vi "f1.vi"() -> ()   [LabVIEW 2026]
uses:
  <vilib>/Analysis/baseanly.llb/Mean (DBL).vi
  <vilib>/numeric/Random Number (Range) DBL.vi
  <vilib>/Analysis/NI_AALBase.lvlib
panel:
  out "opony":cluster{"laps":i32[], dbl[]}[](graph)
  out "zuzycie":cluster{"laps":i32[], dbl[]}[](graph)
  out "czysty":cluster{"laps":i32[], dbl[]}[](graph)
  out "czas":cluster{"laps":i32[], "times":dbl[]}[](graph)
  in  "Porównanie wybranych kierowców\n 2":bool
  in  "kierowca":i32[](listbox)
  out "Error - graph":string
  out "XY Graph 2":cluster{dbl[], dbl[]}(graph)
  in  "wyświetl mapę":bool
  in  "pobierz_kwalifikacje\n 2":bool
  in  "placement":i32[](listbox)
  in  "gp":i32(listbox)
  in  "sezony":i32(listbox)
  in  "pobierz_sezony":bool
  in  "pobierz_gp":bool
  in  "?":enum32{"Sterowanie"}(tab)
  in  "?":bool
  in  "Module path:":path
  in  "Python path:":path
  # "Zanim włączymy progam należy podać siężkę do pythona (wymagana wersja 3.12.x).\n\n     - dla systemu Windows: <dysk>:\\Users\\<użytkownik>\\AppData\\Local\\Programs\\Python\\Python312\n     - dla systemu Mac: /Library/Frameworks/Python.Frameworks/Versions/3.12\n     - dla systemu Linux: /usr/bin/python3 lub /usr/local/bin/python3\n\nPotrzebne biblioteki Pythona, które należy zainsalować przy pomocy pip (bez tworzenia wirtualnego środowiska):\n\n     - urllib3\n\ngdzie:\n     - <dysk>, oznacza dysk główny, na którym znajduje się system \n     - <użytkownik>, nazwa użytkownika\n\nDodatkowo należy podać ścieżkę do modułu, czyli pliku api_F1.py, który znajduje się w folderze z projektem."
  # "Instrukcja obsługi:\n\n1. Pobieranie sezonów, kliknij przycisk \"Pobierz sezony\" — zostanie załadowana lista dostępnych sezonów F1.\n2. Pobieranie wyścigów GP, wybierz sezon z listy, a następnie kliknij przycisk \"Pobierz GP\" — wyświetli się lista Grand Prix dla danego sezonu. \n3. Pobieranie kwalifikacji, kliknij przycisk \"Pobierz kwalifikacje\" — zostaną wyświetleni kierowcy i ich wyniki z kwalifikacji.\n4. Wyświetlanie mapy toru, kliknij przycisk \"Pokaż mapę wybranego GP\" — na ekranie pojawi się schemat toru.\n\nUwaga: Jeśli mapa dla wybranego wyścigu nie istnieje w bazie danych, wyświetli się komunikat informacyjny pod przyciskiem."
  # "Wyniki wybranej kwalifikacji:"
  # "Skórty w wynikach F1:\nDNF - Did Not Finish: nie ukończył\nDNS - Did Not Stat: nie wystartował\nDSQ - Disqualified: dyskwalifikowany\nNC - Not Classified: nie sklasyfikowany\nDNQ - Did Not Qualify: nie zakwalifikował się\nWD - Withdrawn: wycofał się"
  # "Opis i interpretacja wykresów:\n\nCzas okrążeń ( lewy-górny wykres ): \n        - Co przedstawia: Rzeczywisty czas przejechania każdego okrążenia przez kierowcę (w sekundach)\n        - Jak interpretować:\n                  => Spadki - kierowca przyspiesza (nowe opony, mniej paliwa, czsyte okrążenie)\n                  => Wzrosty - kierowca zwalnia (zużyte opony, ruch na torzem obrona pozycji)\n                  => Nagłe piki w górę - pit stop, Safety Car, Virtual Safety Car lub incydent na torze\n                  => Sawtooth (piła) - typowy wzór przy wieloktrotch pitach\n\nCzas \"czysty\" ( prawy-górny wykres ):\n       - Co przedstawia: czas okrążenia po odjęciu wpływu paliwa i opon - teoretyczny czas kierwocy na \"świeżych oponach i z pustym bakiem\"\n       - Jak interpretować: \n                 => Pozwala ocenić czyste tempo kierowcy bez wpływu strategii\n                 => Spadki - kierowca jedzie coraz szybciej (zyskuje doświadczenie w wyścigu, poprawia linie)\n                 => Wzrosty - kierowca ma problem (ruch na torze, błędy, uszkodzenia)\n                 => Prównanie z rzeczystiwtym czasem - różnica pokazuje, ile stracił przez strategię (paliwo + opony)\n\nZużycie paliwa ( lewy-dolny wykres ):\n       - Co przedstawia: Ilość paliwa pozostałego w baku w każdym momencie wyścigu (w kg)\n       - Jak interpretować: \n                 => Linia malejąca - im mniej paliwa, tym lżejszy bolid\n                 => Małe wahania - różnice w zużyciu wynikające z tempa jazdy (szybciej = więcej paliwa)\n                  \nNotka: Zużycie paliwa jest symulowane na podstawie założonego modelu (start z pełnym bakiem ok. 100L, liniowe lub niemal liniowe zużycie z niewielkimi losowymi wahaniami). Nie są to rzeczywiste dane telemetryczne z bolidu.\n\nZyżycie opon ( prawy-dolny wykres ):\n       - Co przedstawia: skumulowana strata czasowa wynikająca z degreadacji opon (w sekundach)\n       - Jak interpretować: \n                 => Odcinki rosnące - opony się zużywają, bolid traci przyczepność i jest wolniejszy\n                 => Spadki do zera - moment wymiany opon w pit stopie (reset zużycia)\n                 => Nachylenie krzywej - szybkość degradacji (im stromiej, tym szybciej opony tracą przyczepność)\n\nNotka: Zyżycie opon jest symulowane (model liniowy z resetem przy pit stopie). W rzeczywistości degradacja zależy od typu opon, temperatury, stylu jazdy i charakterystyki toru - model upraszcza te zależność do stałej straty na okrążenie"
  # "Jeżeli program przestanie odpowiadać, zatnie się lub nic nie będzie się wyświetlało przez dłuższy czas należy zrestartować projekt."
  # "Uwaga techniczna: W przypadku porównania wielu kierowców każdy kierowca rysowany jest na osobnym plocie. Numer plotu zaczyna się od 0 — plot 0 to pierwszy kierowca, plot 1 to drugi kierowca itd. Property Node Active Plot oraz Plot.Name \nmogą powodować błąd — w około 50% przypadków powodowały błąd Invalid property value (Hex 0x435), niezależnie od ustawienia Plots[].Size. Jeżeli pojawi się błąd z tym związany należy kliknąć \"Continue\" do momentu nieskończenia się powiadomień."
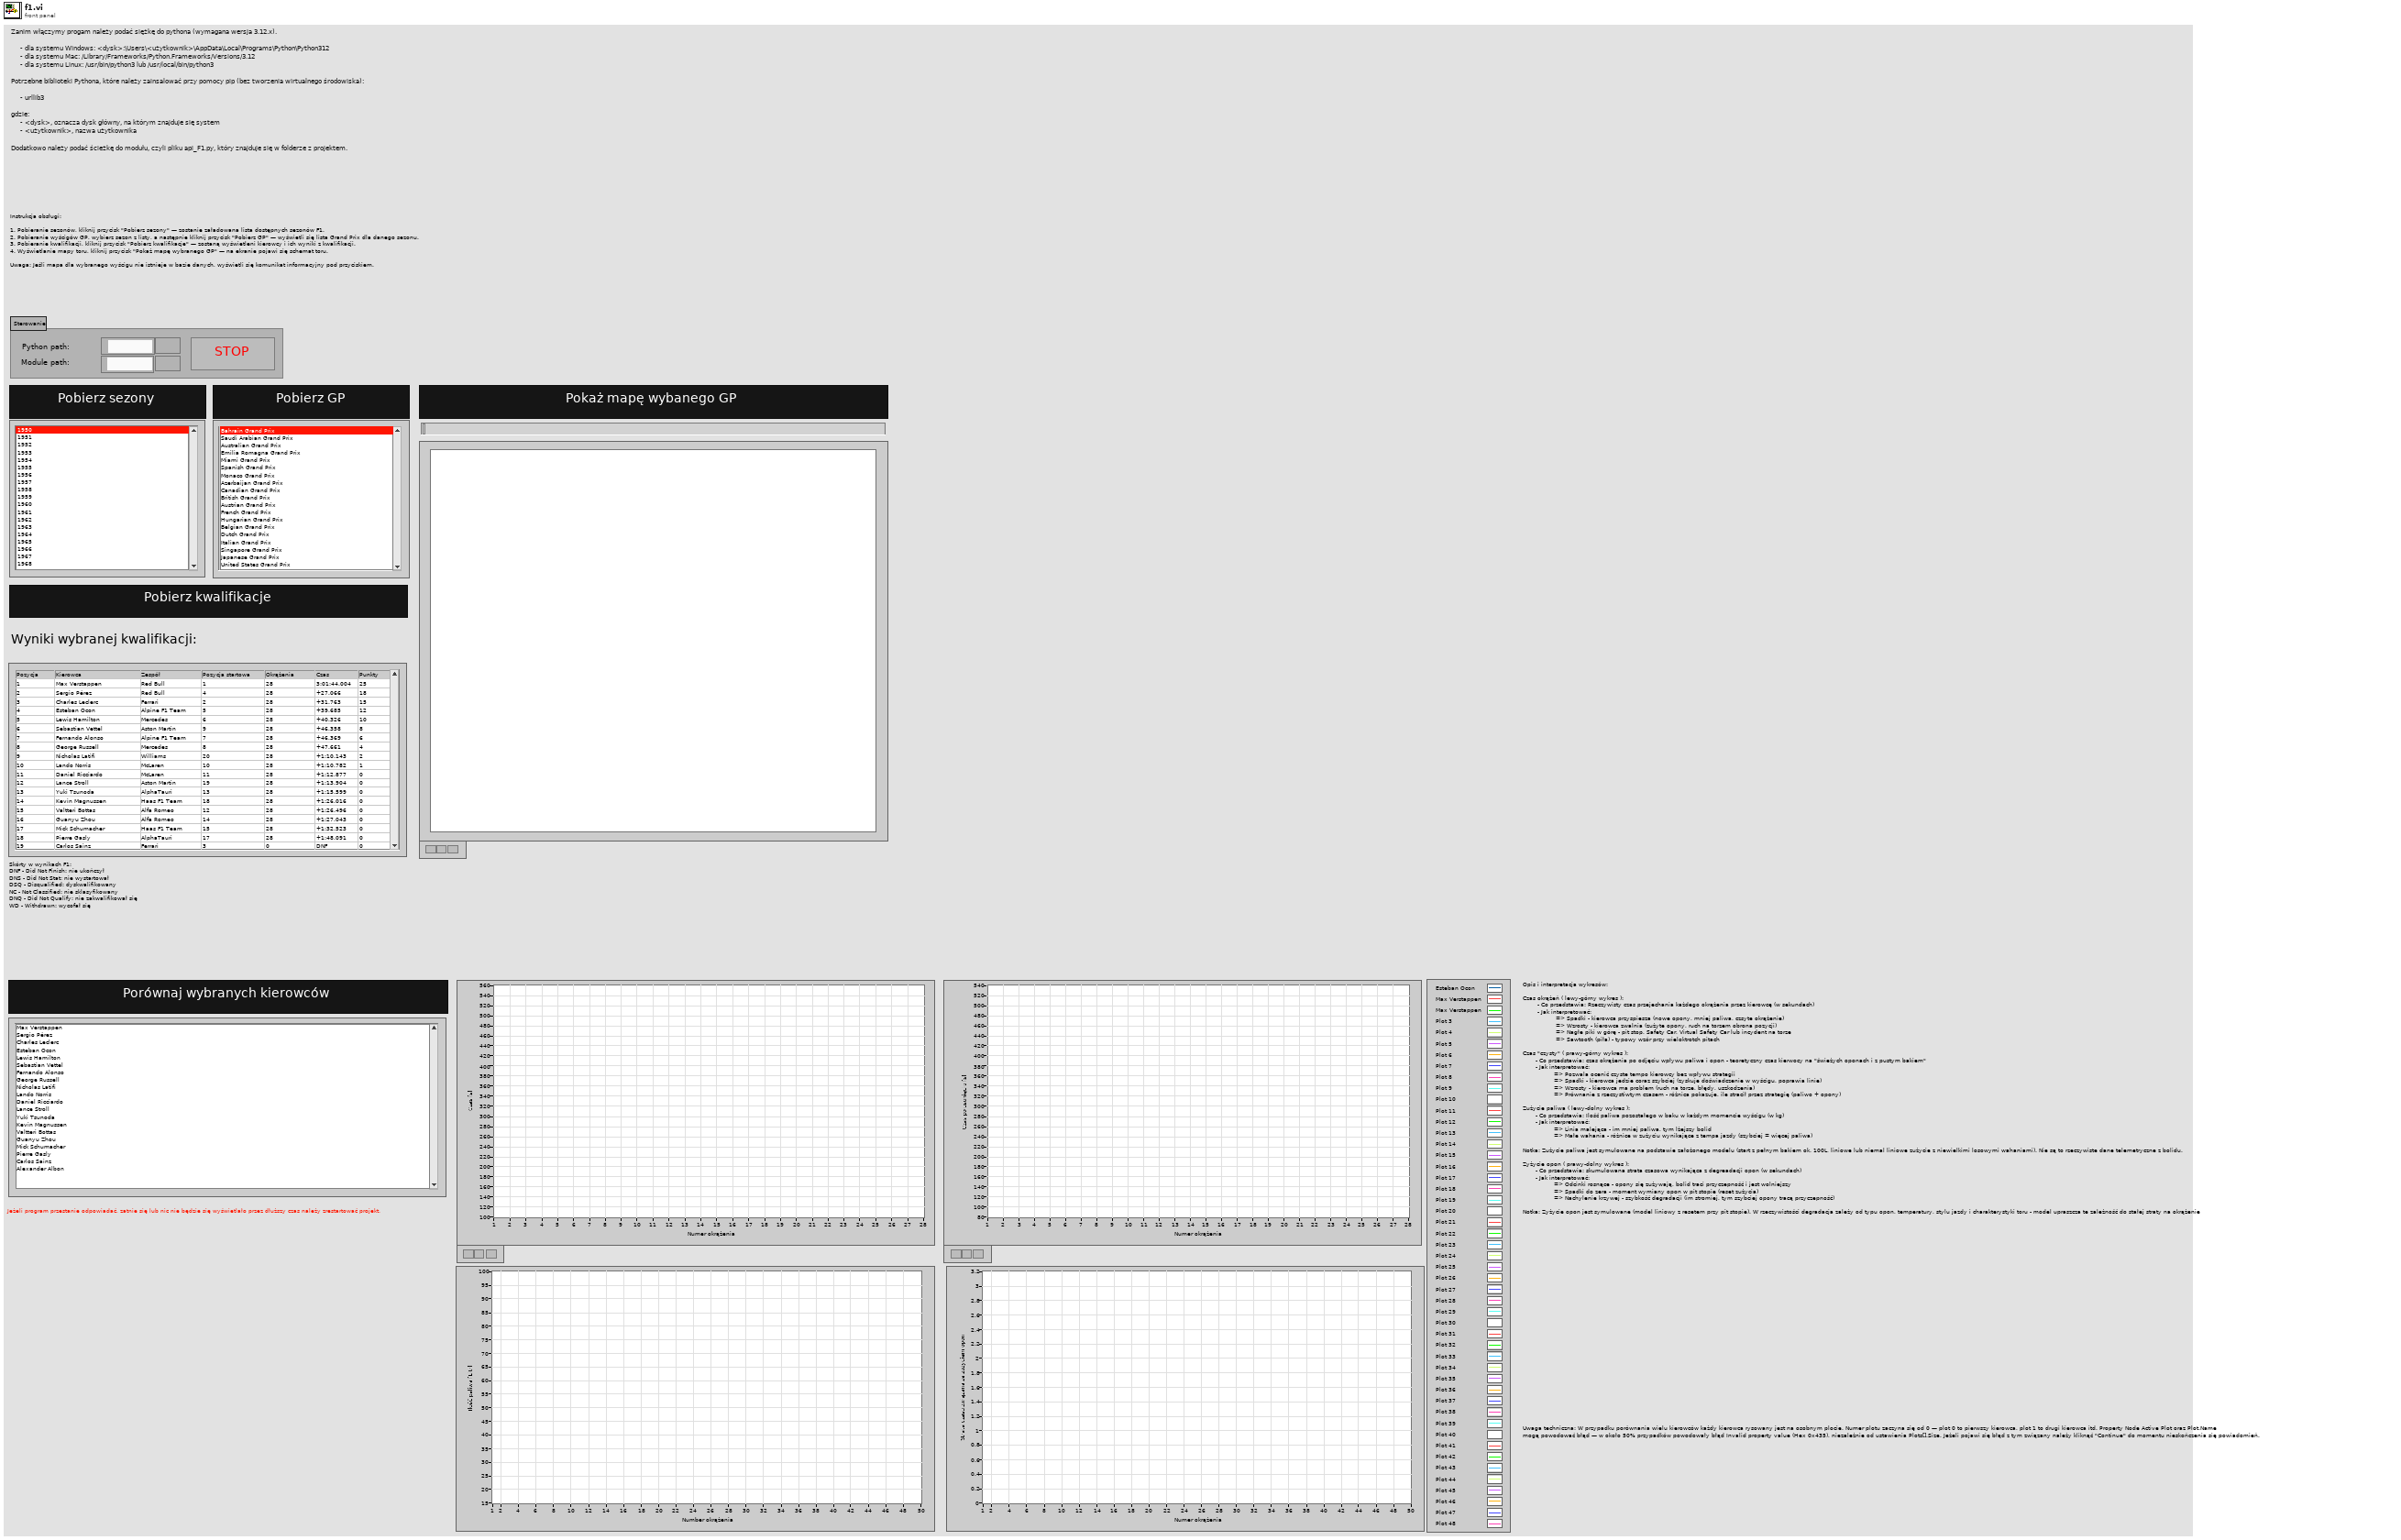
[diagram p1: front panel]
types:
  T1 = cluster{"error":string, "laps":i32[], "times":dbl[], "pits":i32[]}
  T2 = cluster{"position":string, "driver":string, "team":string, "grid":string, "laps":string, "time":string, "points":string}[]
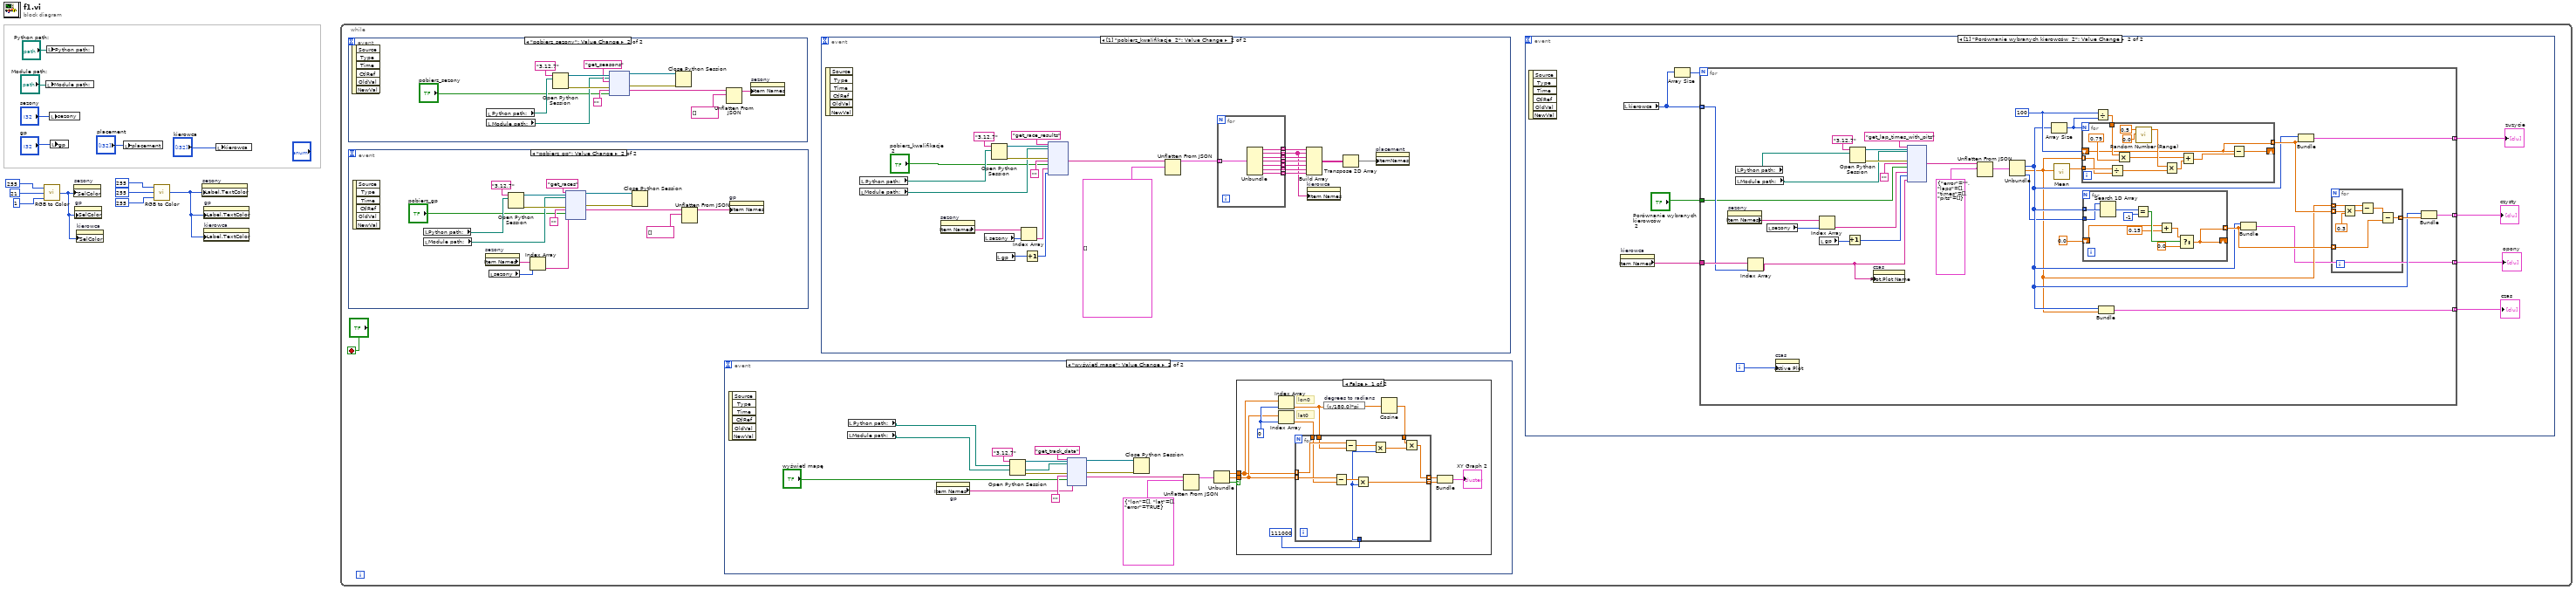
[diagram p0: block diagram]
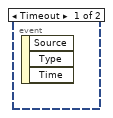
[diagram p2: hidden frame]
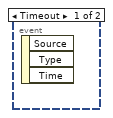
[diagram p3: hidden frame]
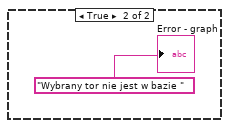
[diagram p4: hidden frame]
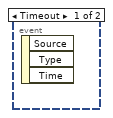
[diagram p5: hidden frame]
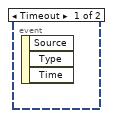
[diagram p6: hidden frame]
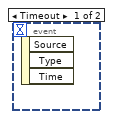
[diagram p7: hidden frame]
diagram:
  n1 = call <vilib>:"RGB to Color.vi"("B"=u8 1, "G"=u8 21, "R"=u8 255) -> ("Color"=w5:u32)
  n2 = local write "Module path:"("Module path:") -> ()
  n3 = local write "Python path:"("Python path:") -> ()
  n4 = local write "sezony"("sezony") -> ()
  n5 = local write "gp"("gp") -> ()
  n6 = property on="sezony" class="LstBox (strict)"("SelColor"=w5) -> ()  [unwired: 2 in, 2 out]
  n7 = property on="gp" class="LstBox (strict)"("SelColor"=w5) -> ()  [unwired: 2 in, 2 out]
  n8 = property on="kierowca" class="LstBox (strict)"("SelColor"=w5) -> ()  [unwired: 2 in, 2 out]
  n9 = local write "placement"("placement") -> ()
  n10 = call <vilib>:"RGB to Color.vi"("B"=u8 255, "G"=u8 255, "R"=u8 255) -> ("Color"=w1:u32)
  n11 = property on="sezony" class="LstBox (strict)"("Label.TextColor"=w1) -> ()  [unwired: 2 in, 2 out]
  n12 = property on="gp" class="LstBox (strict)"("Label.TextColor"=w1) -> ()  [unwired: 2 in, 2 out]
  n13 = property on="kierowca" class="LstBox (strict)"("Label.TextColor"=w1) -> ()  [unwired: 2 in, 2 out]
  n14 = local write "kierowca"("kierowca") -> ()
  n15 = while {
    stop <- "?" stop-if-true
    n16 = event shown="[1] \"pobierz_sezony\": Value Change" {
      selector: _ -> [_ _]
      dyn-events: _ -> [_ _]
      timeout: _ -> [_ _]
      event Timeout {
        n17 = event-data() -> ()  [unwired: 1 in, 3 out]
      }
      event "pobierz_sezony": Value Change {
        n18 = event-data() -> ()  [unwired: 1 in, 6 out]
        n19 = local read "Python path:"() -> (w183:path)
        n20 = local read "Module path:"() -> (w182:path)
        n21 = Open Python Session(python version="3.12.7" ("Python version"), python path=w183) -> (session out=w187:refnum<k35>, error out=w188:errorcluster)  [unwired: 1 in]
        n22 = node ("Python Node")(w187, w182, "get_seasons" ("function name"), w188, "", "pobierz_sezony") -> (w189:refnum<k35>, w190:errorcluster, w178:string)  [unwired: 1 in, 2 out]
        n23 = Close Python Session(session in=w189, error in=w190) -> ()  [unwired: 1 out]
        n24 = Unflatten From JSON(JSON string=w178, type and defaults=string[] []) -> (value=w181:string[])  [unwired: 5 in, 1 out]
        n25 = property on="sezony" class="LstBox (strict)"("Item Names"=w181) -> ()  [unwired: 2 in, 2 out]
      }
    }
    n26 = event shown="[1] \"pobierz_gp\": Value Change" {
      selector: _ -> [_ _]
      dyn-events: _ -> [_ _]
      timeout: _ -> [_ _]
      event Timeout {
        n27 = event-data() -> ()  [unwired: 1 in, 3 out]
      }
      event "pobierz_gp": Value Change {
        n28 = event-data() -> ()  [unwired: 1 in, 6 out]
        n29 = local read "Python path:"() -> (w168:path)
        n30 = local read "Module path:"() -> (w167:path)
        n31 = property on="sezony" class="LstBox (strict)"() -> ("Item Names"=w166:string[])  [unwired: 2 in, 2 out]
        n32 = local read "sezony"() -> (w163:i32)
        n33 = Open Python Session(python version="3.12.7" ("Python version"), python path=w168) -> (session out=w174:refnum<k35>, error out=w175:errorcluster)  [unwired: 1 in]
        n34 = Index Array(array=w166, index=w163) -> (element=w165:string)
        n35 = node ("Python Node")(w174, w167, "get_races" ("function name"), w175, "", "pobierz_gp", w165) -> (w176:refnum<k35>, w177:errorcluster, w164:string)  [unwired: 2 in, 2 out]
        n36 = Close Python Session(session in=w176, error in=w177) -> ()  [unwired: 1 out]
        n37 = Unflatten From JSON(JSON string=w164, type and defaults=string[] []) -> (value=w169:string[])  [unwired: 5 in, 1 out]
        n38 = property on="gp" class="LstBox (strict)"("Item Names"=w169) -> ()  [unwired: 2 in, 2 out]
      }
    }
    n39 = event shown="[1] \"wyświetl mapę\": Value Change" {
      selector: _ -> [_ _]
      dyn-events: _ -> [_ _]
      timeout: _ -> [_ _]
      event Timeout {
        n40 = event-data() -> ()  [unwired: 1 in, 3 out]
      }
      event "wyświetl mapę": Value Change {
        n41 = event-data() -> ()  [unwired: 1 in, 6 out]
        n42 = local read "Module path:"() -> (w95:path)
        n43 = local read "Python path:"() -> (w96:path)
        n44 = property on="gp" class="LstBox (strict)"() -> ("Item Names"=w97:string[])  [unwired: 2 in, 2 out]
        n45 = Open Python Session(python version="3.12.7" ("Python version"), python path=w96) -> (session out=w102:refnum<k35>, error out=w103:errorcluster)  [unwired: 1 in]
        n46 = node ("Python Node")(w102, w95, "get_track_data" ("function name"), w103, "", "wyświetl mapę", w97) -> (w104:refnum<k35>, w105:errorcluster, w94:string)  [unwired: 2 in, 2 out]
        n47 = Close Python Session(session in=w104, error in=w105) -> ()  [unwired: 1 out]
        n48 = Unflatten From JSON(JSON string=w94, type and defaults=cluster{"lon":dbl[], "lat":dbl[], "error":bool} {"lon"=[], "lat"=[], "error"=TRUE}) -> (value=w93:cluster{"lon":dbl[], "lat":dbl[], "error":bool})  [unwired: 5 in, 1 out]
        n49 = Unbundle(w93) -> ("lon"=w89:dbl[], "lat"=w90:dbl[], "error"=w91:bool)
        n50 = case shown="False" w91 {
          tunnel: w90 -> [w114 _]
          tunnel: w89 -> [w113 _]
          frame False {
            w116 = 0 ("index")
            # "lon0"
            # "lat0"
            n51 = Index Array(array=w113, index=w116) -> (element=w112:dbl)
            n52 = Index Array(array=w114, index=w116) -> (element=w109:dbl)
            n53 = expression code="(x/180.0)*pi" "degrees to radians"(w112) -> (w115:dbl)
            n54 = Cosine(x=w115) -> (cos(x)=w110:dbl)
            n55 = for {
              tunnel: w114 -> [w121] mode=indexing
              tunnel: w113 -> [w127] mode=indexing
              tunnel: w112 -> [w126]
              tunnel: 111000 -> [w118]
              tunnel: w110 -> [w123]
              tunnel: [w122] -> w107 mode=indexing
              tunnel: w109 -> [w120]
              tunnel: [w117] -> w108 mode=indexing
              n56 = Subtract(x=w121, y=w120) -> (x-y=w119:dbl)
              n57 = Subtract(x=w127, y=w126) -> (x-y=w125:dbl)
              n58 = Multiply(x=w119, y=w118) -> (x*y=w117:dbl)
              n59 = Multiply(x=w125, y=w118) -> (x*y=w124:dbl)
              n60 = Multiply(x=w123, y=w124) -> (x*y=w122:dbl)
            }
            n61 = Bundle(w107, w108) -> (→"XY Graph 2":cluster{dbl[], dbl[]})  [unwired: 1 in]
          }
          frame True {
            "Error - graph" <- "Wybrany tor nie jest w bazie " ("Error - graph")
          }
        }
      }
    }
    n62 = event shown="[1] \"pobierz_kwalifikacje  2\": Value Change" {
      selector: _ -> [_ _]
      dyn-events: _ -> [_ _]
      timeout: _ -> [_ _]
      event Timeout {
        n63 = event-data() -> ()  [unwired: 1 in, 3 out]
      }
      event "pobierz_kwalifikacje\n 2": Value Change {
        n64 = event-data() -> ()  [unwired: 1 in, 6 out]
        n65 = local read "Module path:"() -> (w130:path)
        n66 = local read "Python path:"() -> (w131:path)
        n67 = property on="sezony" class="LstBox (strict)"() -> ("Item Names"=w147:string[])  [unwired: 2 in, 2 out]
        n68 = local read "sezony"() -> (w148:i32)
        n69 = Open Python Session(python version="3.12.7" ("Python version"), python path=w131) -> (session out=w152:refnum<k35>, error out=w153:errorcluster)  [unwired: 1 in]
        n70 = local read "gp"() -> (w143:i32)
        n71 = Index Array(array=w147, index=w148) -> (element=w146:string)
        n72 = Increment(x=w143) -> (x+1=w144:i32)
        n73 = node ("Python Node")(w152, w130, "get_race_results" ("function name"), w153, "", "pobierz_kwalifikacje\n 2", w146, w144) -> (w134:string)  [unwired: 3 in, 4 out]
        n74 = Unflatten From JSON(JSON string=w134, type and defaults=T2 []) -> (value=w142:T2)  [unwired: 5 in, 1 out]
        n75 = for {
          tunnel: w142 -> [w161] mode=indexing
          tunnel: [w160] -> w141 mode=indexing
          tunnel: [w159] -> w132 mode=indexing
          tunnel: [w158] -> w140 mode=indexing
          tunnel: [w157] -> w139 mode=indexing
          tunnel: [w156] -> w138 mode=indexing
          tunnel: [w155] -> w137 mode=indexing
          tunnel: [w154] -> w136 mode=indexing
          n76 = Unbundle(w161) -> ("position"=w160:string, "driver"=w159:string, "team"=w158:string, "grid"=w157:string, "laps"=w156:string, "time"=w155:string, "points"=w154:string)
        }
        n77 = Build Array(w141, w132, w140, w139, w138, w137, w136) -> (w133:string[][])
        n78 = property on="kierowca" class="LstBox (strict)"("Item Names"=w132) -> ()  [unwired: 2 in, 2 out]
        n79 = Transpose 2D Array(2D array=w133) -> (transposed array=w135:string[][])
        n80 = property on="placement" class="MCListbox (strict)"("ItemNames"=w135) -> ()  [unwired: 2 in, 2 out]
      }
    }
    n81 = event shown="[1] \"Porównanie wybranych kierowców  2\": Value Change" {
      selector: _ -> [_ _]
      dyn-events: _ -> [_ _]
      timeout: _ -> [_ _]
      event Timeout {
        n82 = event-data() -> ()  [unwired: 1 in, 3 out]
      }
      event "Porównanie wybranych kierowców\n 2": Value Change {
        n83 = event-data() -> ()  [unwired: 1 in, 6 out]
        n84 = property on="kierowca" class="LstBox (strict)"() -> ("Item Names"=w23:string[])  [unwired: 2 in, 2 out]
        n85 = local read "kierowca"() -> (w21:i32[])
        n86 = Array Size(array=w21) -> (size(s)=w20:i32)
        n87 = for {
          N: w20 -> [_]
          tunnel: w23 -> [w58]
          tunnel: w21 -> [w57] mode=indexing
          tunnel: "Porównanie wybranych kierowców\n 2" -> [w30]
          tunnel: [w29] -> w19 mode=indexing
          tunnel: [w28] -> w18 mode=indexing
          tunnel: [w27] -> w17 mode=indexing
          tunnel: [w26] -> w16 mode=indexing
          i -> [w25]
          w38 = 100
          n88 = property on="sezony" class="LstBox (strict)"() -> ("Item Names"=w48:string[])  [unwired: 2 in, 2 out]
          n89 = local read "Python path:"() -> (w51:path)
          n90 = local read "Module path:"() -> (w50:path)
          n91 = Index Array(array=w58, index=w57) -> (element=w24:string)
          n92 = local read "sezony"() -> (w49:i32)
          n93 = property on="czas" class="XYGraph (strict)"("Active Plot"=w25) -> ()  [unwired: 2 in, 2 out]
          n94 = Index Array(array=w48, index=w49) -> (element=w47:string)
          n95 = local read "gp"() -> (w46:i32)
          n96 = Increment(x=w46) -> (x+1=w45:i32)
          n97 = Open Python Session(python version="3.12.7" ("Python version"), python path=w51) -> (session out=w55:refnum<k35>, error out=w56:errorcluster)  [unwired: 1 in]
          n98 = property on="czas" class="XYGraph (strict)"("Plot.Plot Name"=w24) -> ()  [unwired: 2 in, 2 out]
          n99 = node ("Python Node")(w55, w50, "get_lap_times_with_pits" ("function name"), w56, "", w30, w47, w45, w24) -> (w41:string)  [unwired: 4 in, 4 out]
          n100 = Unflatten From JSON(JSON string=w41, type and defaults=T1 {"error"="", "laps"=[], "times"=[], "pits"=[]}) -> (value=w43:T1)  [unwired: 5 in, 1 out]
          n101 = Unbundle(w43) -> ("laps"=w33:i32[], "times"=w31:dbl[], "pits"=w32:i32[])  [unwired: 1 out]
          n102 = Array Size(array=w33) -> (size(s)=w39:i32)
          n103 = call-poly <vilib>:"Mean.vi"("X"=w31) -> ("mean"=w37:dbl)  [unwired: 1 out]
          n104 = for {
            shift-right: [w66] -> _
            shift-left: 0.0 -> [w71]
            tunnel: w33 -> [w75] mode=indexing
            tunnel: w32 -> [w67]
            tunnel: [w66] -> w35 mode=indexing
            n105 = Search 1D Array(1D array=w67, element=w75) -> (index of element=w68:i32)  [unwired: 1 in]
            n106 = Equal?(x=w68, y=-1) -> (x = y?=w73:bool)
            n107 = Add(x=w71, y=0.15) -> (x+y=w72:dbl)
            n108 = Select(t=w72, s=w73, f=0.0) -> (s? t:f=w66:dbl)
          }
          n109 = Divide(x=w38, y=w39) -> (x/y=w40:dbl)
          n110 = for {
            N: w39 -> [_]
            tunnel: w40 -> [w79]
            shift-right: [w86] -> _
            shift-left: w38 -> [w76]
            tunnel: w37 -> [w84]
            tunnel: w31 -> [w83] mode=indexing
            tunnel: [w76] -> w36 mode=indexing
            n111 = Divide(x=w84, y=w83) -> (x/y=w80:dbl)
            n112 = Multiply(x=w79, y=0.79) -> (x*y=w77:dbl)
            n113 = call-poly <vilib>:"Random Number (Range).vi"("lower bound (0)"=0.0, "upper bound (100)"=0.5) -> ("number"=w85:dbl)  [unwired: 9 in]
            n114 = Multiply(x=w85, y=w80) -> (x*y=w82:dbl)
            n115 = Add(x=w77, y=w82) -> (x+y=w81:dbl)
            n116 = Subtract(x=w76, y=w81) -> (x-y=w86:dbl)
          }
          n117 = Bundle("laps"=w33, "times"=w31) -> (w28:cluster{"laps":i32[], "times":dbl[]})  [unwired: 1 in]
          n118 = Bundle("laps"=w33, w35) -> (w27:cluster{"laps":i32[], dbl[]})  [unwired: 1 in]
          n119 = Bundle("laps"=w33, w36) -> (w26:cluster{"laps":i32[], dbl[]})  [unwired: 1 in]
          n120 = for {
            tunnel: w31 -> [w65] mode=indexing
            tunnel: w36 -> [w61] mode=indexing
            tunnel: w35 -> [w63] mode=indexing
            tunnel: [w62] -> w34 mode=indexing
            n121 = Multiply(x=w61, y=0.3) -> (x*y=w60:dbl)
            n122 = Subtract(x=w65, y=w60) -> (x-y=w64:dbl)
            n123 = Subtract(x=w64, y=w63) -> (x-y=w62:dbl)
          }
          n124 = Bundle("laps"=w33, w34) -> (w29:cluster{"laps":i32[], dbl[]})  [unwired: 1 in]
        }
        "czysty" <- w19
        "czas" <- w18
        "opony" <- w17
        "zuzycie" <- w16
      }
    }
  }
